vi "Finish.vi"   [LabVIEW 2018]
doc: "This VI is called just before exiting. It is expected to close I/O refnum, save collected data, etc."
uses:
  refnums.vi
types:
  T1 = typedef "WPI_PotentiometerDevRef.ctl" = cluster{"DevStatus":errorcluster, "Analog Channel":T2, "Invert Output":bool}
  T2 = typedef "FPGA_AIChannel.ctl" = enum8{"AI 0", "AI 1", "AI 2", "AI 3", "AI MXP 0", "AI MXP 1", "AI MXP 2", "AI MXP 3", "Invalid"}
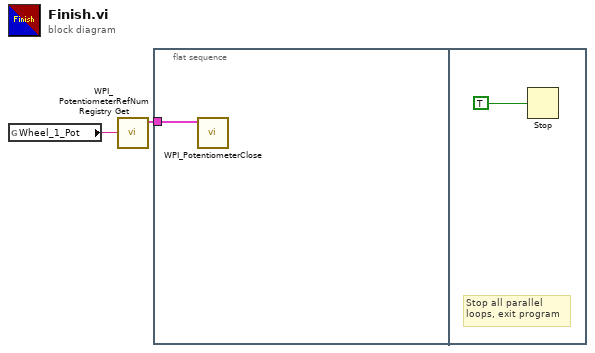
[diagram p0: block diagram]
diagram:
  n1 = global read "refnums.vi" "Wheel_1_Pot"() -> (w2:string)
  n2 = call <vilib>:"WPI_PotentiometerRefNum Registry Get.vi"("refnum name"=w2) -> ("PotDevRef"=w1:T1)  [unwired: 9 in, 1 out]
  n3 = flat-sequence {
    tunnel: w1 -> [w3]
    frame #0 {
      n4 = call <vilib>:"WPI_PotentiometerClose.vi"("PotDevRef"=w3) -> ()  [unwired: 10 in, 1 out]
    }
    frame #1 {
      # "Stop all parallel\nloops, exit program"
      n5 = Stop(stop? (T)=TRUE ("Quit")) -> ()
    }
  }
